vi "Filtr_sumu.vi"(2 "i":i32, 3 "Citlivost 2":i32, 4 "trig_in":bool=TRUE) -> (1 "trig_out":bool=TRUE)   [LabVIEW 2019]
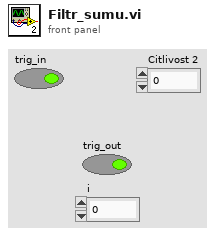
[diagram p1: front panel]
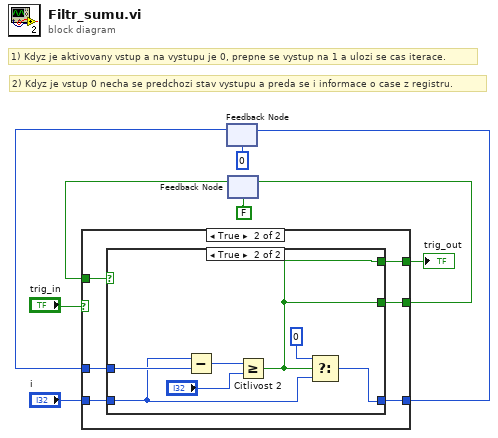
[diagram p0: block diagram]
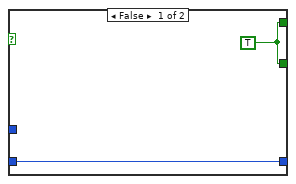
[diagram p3: hidden frame]
diagram:
  # "2) Kdyz je vstup 0 necha se predchozi stav vystupu a preda se i informace o case z registru."
  # "1) Kdyz je aktivovany vstup a na vystupu je 0, prepne se vystup na 1 a ulozi se cas iterace."
  n1 = feedback #1(0 ("i")) -> (w2:i32)
  n2 = feedback #2(FALSE) -> (w4:bool)
  n3 = case shown="True" "trig_in" {
    tunnel: [w11 w17] -> w8
    tunnel: "i" -> [_ w16]
    tunnel: [w10 w15] -> w6
    tunnel: [w11 w14] -> w5
    tunnel: w4 -> [w11 w13]
    tunnel: w2 -> [w10 w12]
    frame False {
    }
    frame True {
      n4 = case shown="True" w13 {
        tunnel: [w18 w24] -> w17
        tunnel: w16 -> [w19 w21]
        tunnel: [w19 w22] -> w15
        tunnel: [w18 w24] -> w14
        tunnel: w12 -> [_ w23]
        frame False {
          w18 = TRUE
        }
        frame True {
          n5 = Subtract(x=w21, y=w23) -> (x-y=w26:i32)
          n6 = Greater Or Equal?(x=w26, y="Citlivost 2") -> (x >= y?=w24:bool)
          n7 = Select(t=0, s=w24, f=w21) -> (s? t:f=w22:i32)
        }
      }
    }
  }
  "trig_out" <- w8
  n8 = feedback-in #1(w6) -> ()
  n9 = feedback-in #2(w5) -> ()
